vi "相对码变绝对码.vi"(1 "相对码":u32[](array[numeric])) -> (0 "绝对码":i32[](array[numeric]))   [LabVIEW 2013]
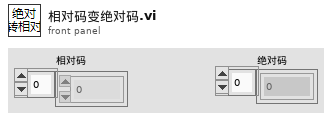
[diagram p1: front panel]
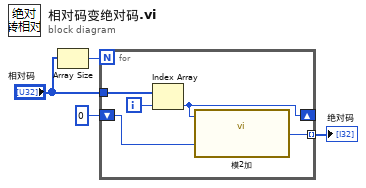
[diagram p0: block diagram]
diagram:
  n1 = Array Size(array="相对码") -> (size(s)=w4:i32)
  n2 = for {
    N: w4 -> [_]
    tunnel: "相对码" -> [w7]
    tunnel: [w9] -> w2 mode=indexing
    shift-right: [w5] -> _
    shift-left: 0 -> [w6]
    i -> [w8]
    n3 = Index Array(array=w7, index=w8) -> (element=w5:u32)
    n4 = call "模2加.vi"("b"=w6, "a"=w5) -> ("c"=w9:u32)
  }
  "绝对码" <- w2
